vi "Access Data Through Reference.vi"(10 "Time Out In ms":i32=-1, 11 "DVR In":refnum<data-value>) -> (0 "Time Out":bool, 2 "Data Out":u16[](array[numeric]), 3 "DVR Out":refnum<data-value>)   [LabVIEW 2019, in "Circular Buffer 1D U16 DVR Queue.lvclass"]
uses:
  Circular Buffer 1D U16 DVR Queue.lvclass
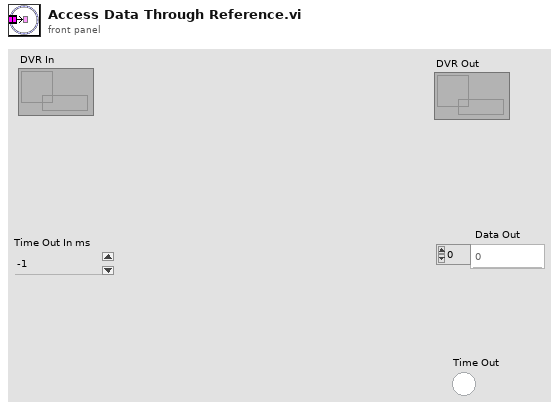
[diagram p1: front panel]
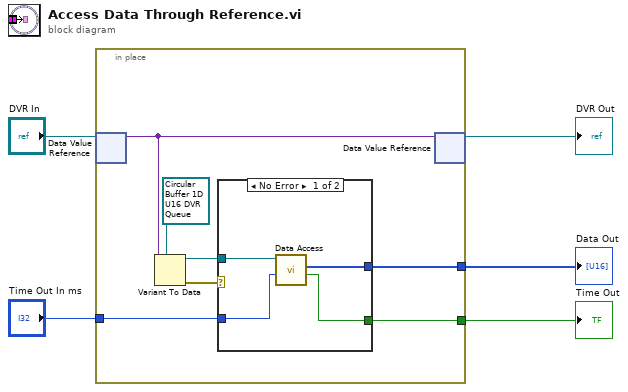
[diagram p0: block diagram]
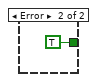
[diagram p2: hidden frame]
diagram:
  n1 = in-place {
    in-place-border: "Time Out In ms" -> [w8]
    in-place-border: [w7] -> w2
    in-place-border: [w6] -> w1
    n2 = in-place-dvr #1("DVR In") -> (w11:variant)  [unwired: 1 out]
    n3 = Variant To Data(type=refnum<class "Circular Buffer 1D U16 DVR Queue.lvclass"> refnum ("Circular Buffer 1D U16 DVR Queue.lvclass"), Variant=w11) -> (data=w9:refnum<class "Circular Buffer 1D U16 DVR Queue.lvclass">, error out=w10:errorcluster)  [unwired: 1 in]
    n4 = case shown="No Error" w10 {
      tunnel: w9 -> [w16 _]
      tunnel: w8 -> [w15 _]
      tunnel: [w14 _] -> w7
      tunnel: [w13 TRUE ("Time Out")] -> w6
      frame No Error {
        n5 = call "Data Access.vi"("Time Out In ms"=w15, "Circular Buffer 1D U16 DVR Queue in"=w16) -> ("Time Out"=w13:bool, "Data Out"=w14:u16[])  [unwired: 7 in, 1 out]
      }
      frame Error {
      }
    }
    n6 = in-place-dvr #1(w11) -> (→"DVR Out":refnum<data-value>)  [unwired: 1 out]
  }
  "Data Out" <- w2
  "Time Out" <- w1
